vi "Configure Calc Smooth.vi"(8 "error in (no error)":errorcluster, 9 "Smoothing Points (10)":dbl=10.0 min=2.0 max=100.0 step=1.0 format="%#_3g", 10 "Calculate Smoothing  (0: Off)":u16(ring) format="%.0g" items=["Off", "On"], 11 "VISA resource name":refnum<visa-resource-name>) -> (0 "error out":errorcluster, 3 "VISA resource name out":refnum<visa-resource-name>)   [LabVIEW 2017, in "ADCMT7451_ADC.lvlib"]
doc: "Enables or disables smoothing calculation."
uses:
  ADCMT7451_ADC.lvlib
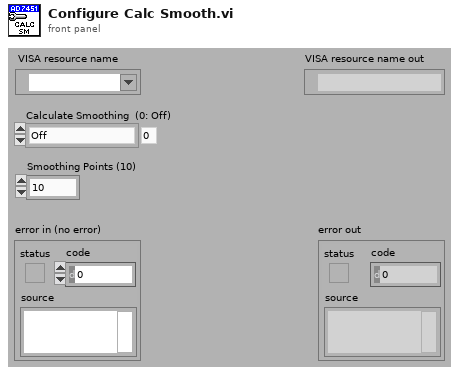
[diagram p1: front panel]
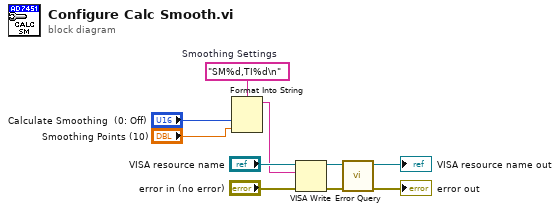
[diagram p0: block diagram]
diagram:
  w4 = "SM%d,TI%d\n"  # Smoothing Settings
  n1 = Format Into String(format string=w4, "Calculate Smoothing  (0: Off)", "Smoothing Points (10)") -> (resulting string=w1:string)  [unwired: 2 in, 1 out]
  n2 = VISA Write(VISA resource name="VISA resource name", write buffer=w1, error in (no error)="error in (no error)") -> (VISA resource name out=w6:refnum<visa-resource-name>, error out=w5:errorcluster)  [unwired: 1 out]
  n3 = call "Error Query.vi"("error in (no error)"=w5, "VISA resource name"=w6) -> ("error out"=→"error out":errorcluster, "VISA resource name out"=→"VISA resource name out":refnum<visa-resource-name>)  [unwired: 6 in, 2 out]
